vi "文件重命名减1.vi"(9 "名称或相对路径":string, 11 "源路径":path) -> ()   [LabVIEW 2016, in "数据传输系统-04.lvlib" / "自动更新.lvlib" / "TCP文件传输系统.lvlib" / "TCP接收文件.lvlib"]
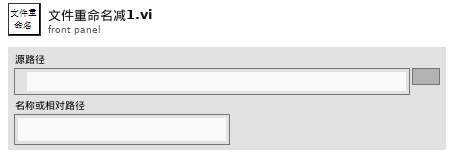
[diagram p1: front panel]
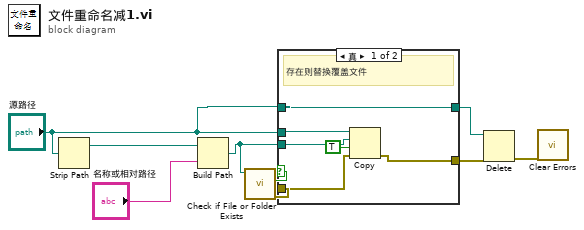
[diagram p0: block diagram]
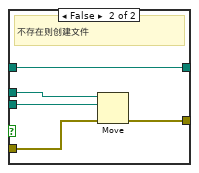
[diagram p2: hidden frame]
diagram:
  n1 = Strip Path(path="源路径") -> (stripped path=w9:path)  [unwired: 1 out]
  n2 = Build Path(base path=w9, name or relative path="名称或相对路径") -> (appended path=w6:path)
  n3 = call <vilib>:"Check if File or Folder Exists.vi"("path"=w6) -> ("error out"=w2:errorcluster, "file or folder exists?"=w7:bool)  [unwired: 8 in, 1 out]
  n4 = case shown="真" w7 {
    tunnel: "源路径" -> [w14 w20]
    tunnel: w6 -> [w13 w19]
    tunnel: "源路径" -> [w15 w18]
    tunnel: [w15 w18] -> w4
    tunnel: [w10 w17] -> w3
    tunnel: w2 -> [w11 w16]
    frame True {
      # "存在则替换覆盖文件"
      n5 = Copy(8:w11, 9:TRUE ("覆盖(F)"), 10:w13, 11:w14) -> (0:w10:errorcluster)  [unwired: 1 in, 2 out]
    }
    frame False {
      # "不存在则创建文件"
      n6 = Move(source path=w20, error in=w16, 10:w19) -> (error out=w17:errorcluster)  [unwired: 2 in, 2 out]
    }
  }
  n7 = Delete(path (use dialog)=w4, error in=w3) -> (error out=w1:errorcluster)  [unwired: 3 in, 2 out]
  n8 = call <vilib>:"Clear Errors.vi"("error in (no error)"=w1) -> ()  [unwired: 5 in, 2 out]
